vi "BRig_RT_getAvgStats.vi"(0 "input_dataCurrent":u16[](array[numeric]), 5 "input_dataBlock":u16[][](array[numeric])) -> (6 "T2R_total":u16, 8 "T2R_avg":dbl, 10 "BTPR_total":u16, 15 "BTPR_avg":dbl)   [LabVIEW 2014]
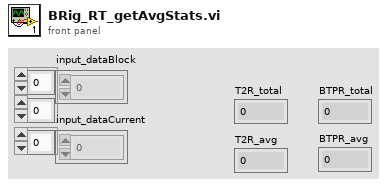
[diagram p1: front panel]
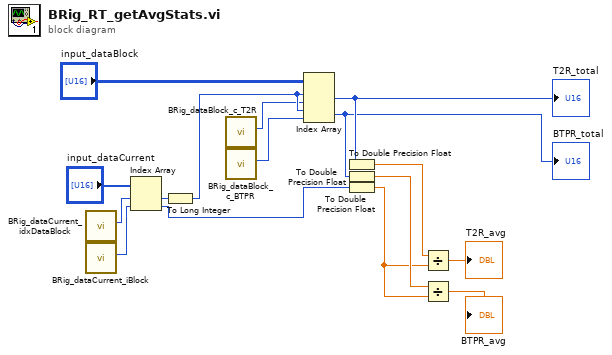
[diagram p0: block diagram]
diagram:
  n1 = call "BRig_dataCurrent_idxDataBlock.vi"() -> ("output_idxDataBlock"=w14:i32)  [unwired: 11 in]
  n2 = call "BRig_dataCurrent_iBlock.vi"() -> ("output_iBlock"=w2:i32)  [unwired: 11 in]
  n3 = Index Array(array="input_dataCurrent", index #1=w14, index #2=w2) -> (element #1=w13:u16, element #2=w1:u16)
  n4 = To Long Integer(number=w13) -> (32bit integer=w12:i32)
  n5 = call "BRig_dataBlock_c_T2R.vi"() -> ("output_c_T2R"=w11:i32)  [unwired: 11 in]
  n6 = call "BRig_dataBlock_c_BTPR.vi"() -> ("output_c_BTPR"=w10:i32)  [unwired: 11 in]
  n7 = Index Array(array="input_dataBlock", index (row) #1=w12, index (col) #1=w11, index (row) #2=w12, index (col) #2=w10) -> (element #1=w9:u16, element #2=w8:u16)
  "T2R_total" <- w9
  "BTPR_total" <- w8
  n8 = To Double Precision Float(number=w9) -> (double precision float=w7:dbl)
  n9 = To Double Precision Float(number=w8) -> (double precision float=w6:dbl)
  n10 = To Double Precision Float(number=w1) -> (double precision float=w5:dbl)
  n11 = Divide(x=w7, y=w5) -> (x/y=→"T2R_avg":dbl)
  n12 = Divide(x=w6, y=w5) -> (x/y=→"BTPR_avg":dbl)
